vi "Port Flush (SubVI).vi"(2 "error in":errorcluster, 3 "VISA Refnum in":refnum<visa-resource-name>) -> (0 "error out":errorcluster, 1 "VISA Refnum out":refnum<visa-resource-name>)   [LabVIEW 2017]
doc: "Try to hard flush the buffer by reading continuously on the COM port until no data is no longer readable.\nMade by Tanguy BOULARD\nTHALES FRANCE"
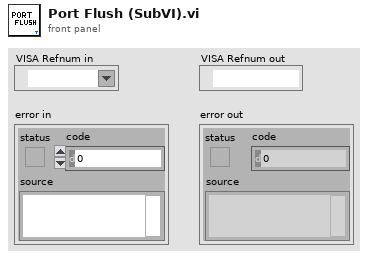
[diagram p1: front panel]
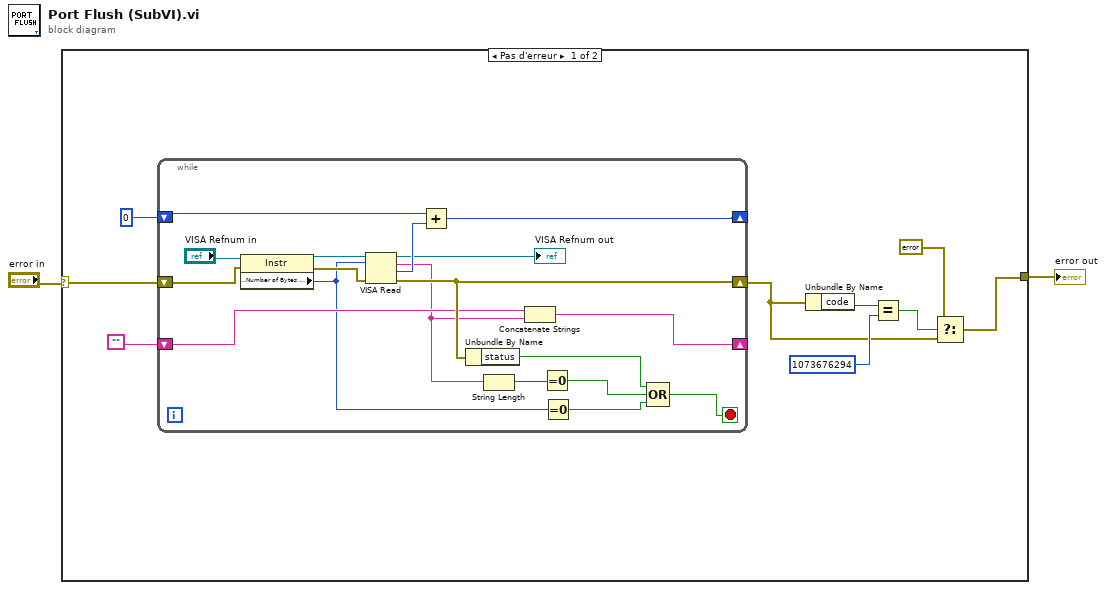
[diagram p0: block diagram]
diagram:
  n1 = case shown="Pas d'erreur" "error in" {
    selector: "error in" -> [w11 w30]
    tunnel: [w3 w30] -> w2
    frame No Error {
      n2 = while {
        shift-right: [w26] -> w4
        shift-left: w11 -> [w21]
        shift-right: [w27] -> _
        shift-left: u32 0 -> [w29]
        shift-right: [w24] -> _
        shift-left: "" -> [w25]
        stop <- w13 stop-if-true
        n3 = property class="Instr"(reference="VISA Refnum in", error in=w21) -> (reference out=w19:refnum<visa-resource-name>, error out=w20:errorcluster, "Serial Settings:Number of Bytes at Serial Port"=w18:u32)
        n4 = VISA Read(VISA resource name=w19, byte count=w18, error in (no error)=w20) -> (VISA resource name out=→"VISA Refnum out":refnum<visa-resource-name>, read buffer=w12:string, return count=w28:u32, error out=w26:errorcluster)
        n5 = Add(x=w29, y=w28) -> (x+y=w27:u32)
        n6 = Unbundle By Name(w26) -> ("status"=w16:bool)
        n7 = String Length(string=w12) -> (length=w17:i32)
        n8 = Concatenate Strings(w25, w12) -> (w24:string)
        n9 = Equal To 0?(x=w17) -> (x = 0?=w15:bool)
        n10 = Equal To 0?(x=w18) -> (x = 0?=w14:bool)
        n11 = Compound Arithmetic op=OR(w16, w15, w14) -> (w13:bool)
      }
      n12 = Unbundle By Name(w4) -> ("code"=w8:i32)
      n13 = Equal?(x=w8, y=1073676294) -> (x = y?=w6:bool)
      n14 = Select(t=errorcluster {"status"=FALSE, "code"=0, "source"=""}, s=w6, f=w4) -> (s? t:f=w3:errorcluster)
    }
    frame Error {
    }
  }
  "error out" <- w2
